vi "GetSetpoint1.vi"(8 "Error In":errorcluster, 11 "Omega CSi32 In":refnum<visa-resource-name>) -> (0 "Error Out":errorcluster, 2 "Setpoint 1 (C)":dbl format="%.1f", 3 "Omega CSi32 Out":refnum<visa-resource-name>)   [LabVIEW 2012, in "Omega-CSi32.lvlib"]
uses:
  Omega-CSi32.lvlib
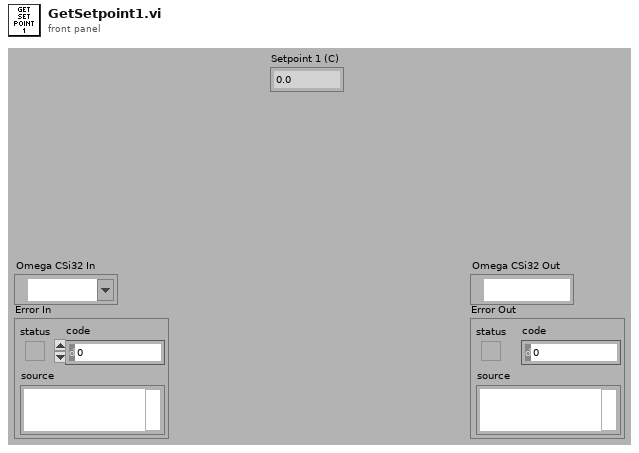
[diagram p1: front panel]
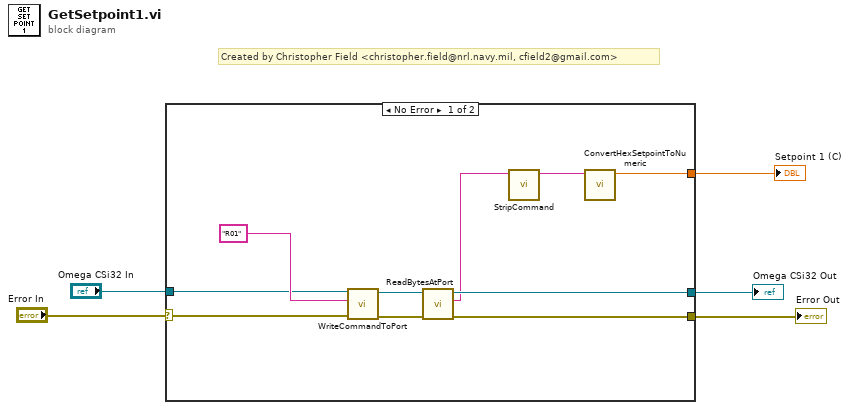
[diagram p0: block diagram]
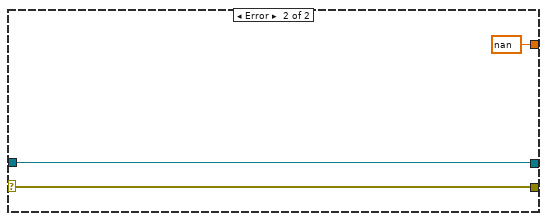
[diagram p2: hidden frame]
diagram:
  # "Created by Christopher Field <christopher.field@nrl.navy.mil, cfield2@gmail.com>"
  n1 = case shown="No Error" "Error In" {
    selector: "Error In" -> [w6 w17]
    tunnel: [w15 nan ("Numeric Setpoint (C)")] -> w5
    tunnel: [w13 w18] -> w4
    tunnel: [w12 w17] -> w3
    tunnel: "Omega CSi32 In" -> [w7 w18]
    frame No Error {
      n2 = call "WriteCommandToPort.vi"("Error In"=w6, "Command"="R01", "Omega CSi32 In"=w7) -> ("Error Out"=w9:errorcluster, "Omega CSi32 Out"=w10:refnum<visa-resource-name>)  [unwired: 7 in]
      n3 = call "ReadBytesAtPort.vi"("Error In"=w9, "Omega CSi32 In"=w10) -> ("Error Out"=w12:errorcluster, "Read Buffer"=w11:string, "Omega CSi32 Out"=w13:refnum<visa-resource-name>)  [unwired: 7 in]
      n4 = call "StripCommand.vi"("Command"=w11) -> ("Stripped Command"=w14:string)  [unwired: 10 in]
      n5 = call "ConvertHexSetpointToNumeric.vi"("Hex Setpoint"=w14) -> ("Numeric Setpoint (C)"=w15:dbl)  [unwired: 10 in]
    }
    frame Error {
    }
  }
  "Omega CSi32 Out" <- w4
  "Error Out" <- w3
  "Setpoint 1 (C)" <- w5
